vi "set configuration by UID.vi"(8 "error in":errorcluster, 9 "configuration":refnum<class "NISE_CEF_serializable configuration.lvclass">, 10 "alias":string, 11 "NISE_CEF_HierarchyRepo in":refnum<class "NISE_CEF_HierarchyRepo.lvclass">) -> (0 "error out":errorcluster, 3 "NISE_CEF_HierarchyRepo out":refnum<class "NISE_CEF_HierarchyRepo.lvclass">)   [LabVIEW 2013, in "NISE_CEF_HierarchyRepo.lvclass"]
uses:
  NISE_CEF_HierarchyRepo.lvclass
  serializable configuration/NISE_CEF_serializable configuration.lvclass
  NISE_CEF_HierarchyRepo.lvclass/NISE_CEF_HierarchyRepo.ctl
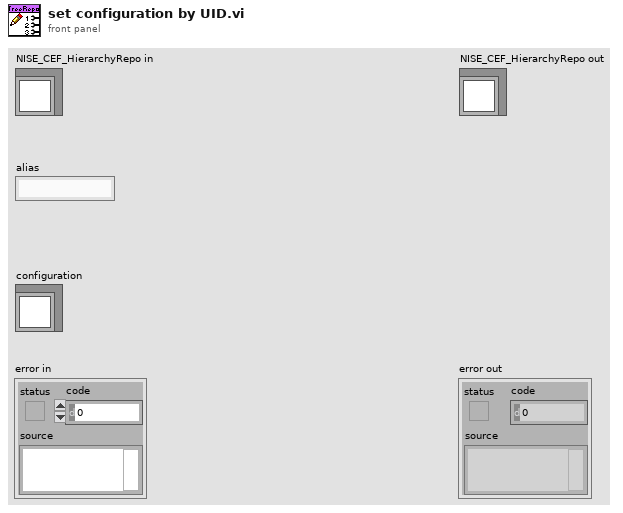
[diagram p1: front panel]
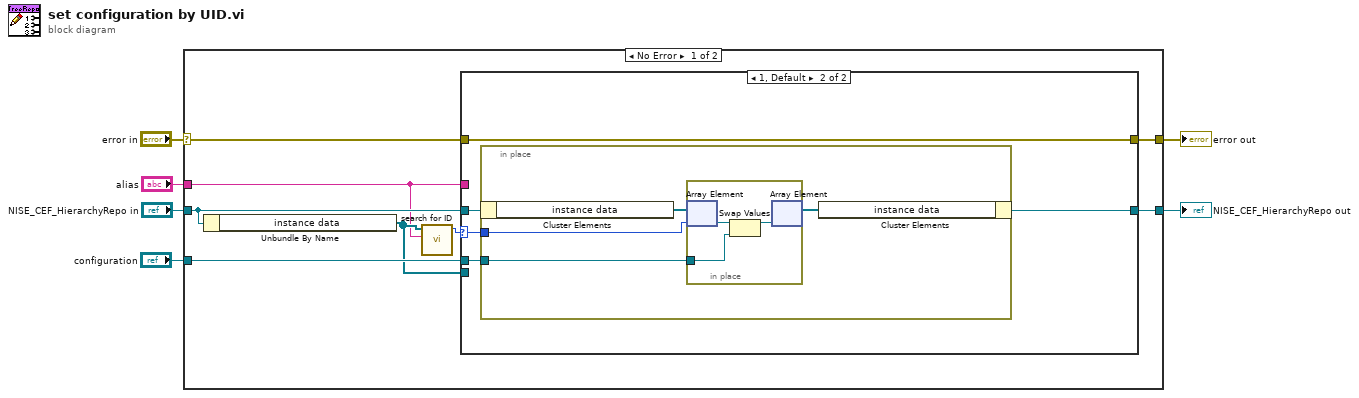
[diagram p0: block diagram]
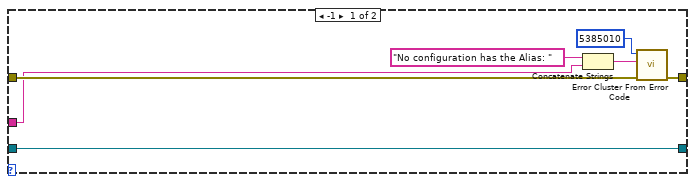
[diagram p2: hidden frame]
diagram:
  n1 = case shown="No Error" "error in" {
    selector: "error in" -> [w14 w35]
    tunnel: [w13 w35] -> w5
    tunnel: [w10 w34] -> w3
    tunnel: "NISE_CEF_HierarchyRepo in" -> [w11 w34]
    tunnel: "alias" -> [w7 _]
    tunnel: "configuration" -> [w12 _]
    frame No Error {
      n2 = Unbundle By Name(w11) -> ("instance data"=w8:refnum<class "NISE_CEF_serializable configuration.lvclass">[])
      n3 = call "search for ID.vi"("instance id"=w7, "instance data"=w8) -> ("index"=w9:i32)  [unwired: 9 in]
      n4 = case shown="1, Default" w9 {
        selector: w9 -> [_ w23]
        tunnel: w8 -> [_ _]
        tunnel: w14 -> [w21 w26]
        tunnel: [w20 w26] -> w13
        tunnel: w7 -> [w17 _]
        tunnel: w12 -> [_ w22]
        tunnel: w11 -> [w15 w25]
        tunnel: [w15 w24] -> w10
        frame -1 {
          n5 = Concatenate Strings("No configuration has the Alias: " ("string"), w17) -> (w18:string)
          n6 = call <vilib>:"Error Cluster From Error Code.vi"("error in (no error)"=w21, "error message (\"\")"=w18, "error code (0)"=5385010) -> ("error out"=w20:errorcluster)  [unwired: 6 in]
        }
        frame 1, Default {
          n7 = in-place {
            in-place-border: w23 -> [w28]
            in-place-border: w22 -> [w27]
            n8 = in-place-cluster #1(w25) -> ("instance data"=w30:refnum<class "NISE_CEF_serializable configuration.lvclass">[])
            n9 = in-place {
              in-place-border: w27 -> [w32]
              n10 = in-place-array #2(w30, w28) -> (w33:refnum<class "NISE_CEF_serializable configuration.lvclass">)
              n11 = Swap Values(12:w33, 14:w32) -> (1:w31:refnum<class "NISE_CEF_serializable configuration.lvclass">)  [unwired: 1 in, 1 out]
              n12 = in-place-array #2(w31) -> (w29:refnum<class "NISE_CEF_serializable configuration.lvclass">[])  [unwired: 1 out]
            }
            n13 = in-place-cluster #1("instance data"=w29) -> (w24:refnum<class "NISE_CEF_HierarchyRepo.lvclass">)
          }
        }
      }
    }
    frame Error {
    }
  }
  "error out" <- w5
  "NISE_CEF_HierarchyRepo out" <- w3
